vi "main_SMU.vi"() -> ()   [LabVIEW 2018]
uses:
  <instrlib>/Keithley 622x LV 2009/Configure/Source/Typedefs/KE622x -- Voltage Limit.ctl
  <instrlib>/Keithley 622x LV 2009/Configure/Output/Typedefs/KE6221 -- Output Response.ctl
  <instrlib>/Keithley 622x LV 2009/Utility/Typedefs/KE622x -- Instrument Type.ctl
  <instrlib>/Keithley 622x LV 2009/Typedefs/KE622x -- On Off Control.ctl
  <instrlib>/Keithley 622x LV 2009/Configure/Source/Typedefs/KE622x -- Current Range.ctl
  <instrlib>/Keithley 622x LV 2009/Configure/Source/Typedefs/KE622x -- Current Ranges.ctl
  <instrlib>/Keithley 622x LV 2009/Configure/Source/Typedefs/KE622x -- Current Level.ctl
  <vilib>/Utility/file.llb/Write Delimited Spreadsheet (string).vi
  <instrlib>/Keithley 622x LV 2009/Keithley 622x.lvlib
  <instrlib>/Keithley 2450/Keithley 2450.lvlib
panel:
  in  "Compliance Level (0.1)":dbl=0.1
  in  "Output Level (0)":dbl
  out "Voltage":sgl[](array[numeric])
  in  "VISA resource name":refnum<visa-resource-name>
  in  "VISA Switch":refnum<visa-resource-name>="GPIB::6"
  out "Close Channel List":string
  in  "Configurations":enum32{"Radio Selection 1", "Radio Selection 2"}(radio)
  out "Iteration number":i32
  out "Current  (A)":dbl
  out "Mean Voltage  (V1-V8)":dbl
  in  "Step Size":T1=0.001 min=-0.105 max=0.105 format="%.4p"
  in  "End":T1=0.001 min=-0.105 max=0.105 format="%.4p"
  in  "Start":T1=0.001 min=-0.105 max=0.105 format="%.4p"
  in  "Turn Off Output If Voltage Limit?":bool=TRUE
  out "Interlock Tripped?":bool
  out "Voltage Limit?":bool
  in  "Check For SCPI Errors? (T)":bool=TRUE
  in  "Current Range In":T2={"Auto Range?"=TRUE, "Man / Selected\nRange"=enum."2nA"}
  in  "Analog Filter State":T4
  in  "Output Response":T5=enum."Slow"
  in  "Voltage Limit (V)":T6=10.0 min=0.1 max=105.0 step=0.01 format="%.2p"
  out "error at Current off":errorcluster
  out "error at current On":errorcluster
  in  "VISA resource dc ac current source (16)":refnum<visa-resource-name>
  out "Configuration Error":errorcluster
  in  "array":dbl[](array[numeric])
  out "output array":dbl[](array[numeric])
  in  "Instrument Type 2":T7=enum."KE6221"
  # "( select : GPIB0::16::INSTR )"
  # "( select : USB0::0x05E6::0x2450::04345639::INSTR )"
  # "( select : USB0::0x05E6::0x3706::04368238::INSTR )"
types:
  T1 = typedef "Keithley 622x.lvlib/KE622x -- Current Level.ctl" = dbl
  T2 = typedef "Keithley 622x.lvlib/KE622x -- Current Range.ctl" = cluster{"Auto Range?":bool, "Man / Selected\nRange":T3}
  T3 = typedef "Keithley 622x.lvlib/KE622x -- Current Ranges.ctl" = enum16{"2nA", "20nA", "200nA", "2uA", "20uA", "200uA", "2mA", "20mA", "100mA"}
  T4 = typedef "Keithley 622x.lvlib/KE622x -- On Off Control.ctl" = enum16{"Off", "On"}
  T5 = typedef "Keithley 622x.lvlib/KE6221 -- Output Response.ctl" = enum16{"Fast", "Slow"}
  T6 = typedef "Keithley 622x.lvlib/KE622x -- Voltage Limit.ctl" = dbl
  T7 = typedef "Keithley 622x.lvlib/KE622x -- Instrument Type.ctl" = enum16{"KE6220", "KE6221"}
  T8 = enum16{"Close", "Close Exclusive", "Close Slot Exclusive", "Open", "Open All"}
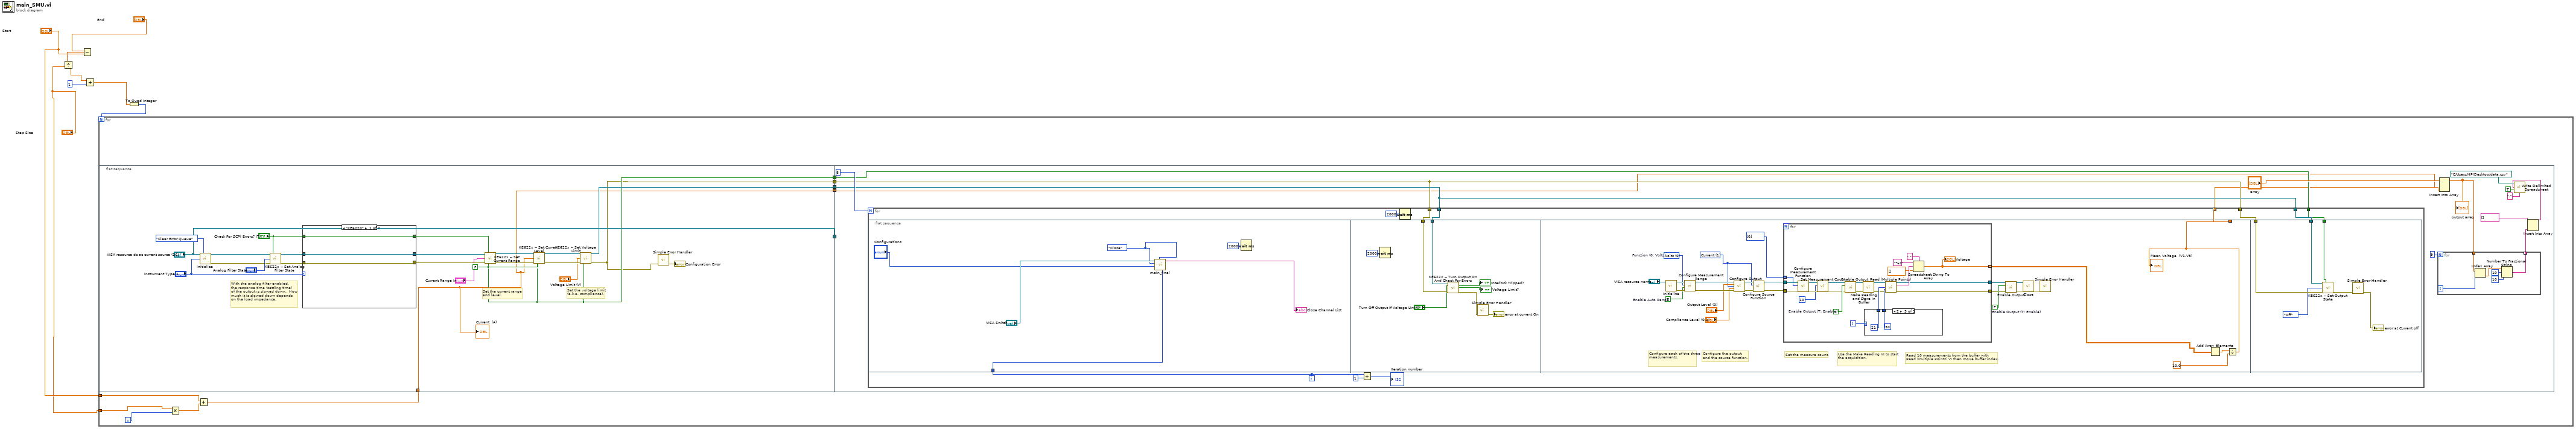
[diagram p0: block diagram]
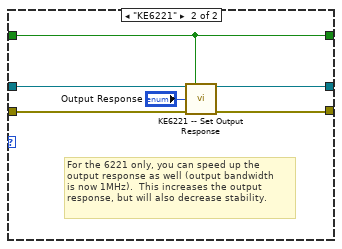
[diagram p2: hidden frame]
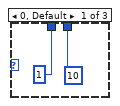
[diagram p3: hidden frame]
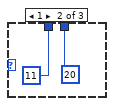
[diagram p4: hidden frame]
diagram:
  n1 = Subtract(x="End", y="Start") -> (x-y=w8:T1)
  n2 = Divide(x=w8, y="Step Size") -> (x/y=w4:T1)
  n3 = Add(x=w4, y=1) -> (x+y=w2:T1)
  n4 = To Quad Integer(1:w2) -> (0:w1:i64)
  n5 = for {
    N: w1 -> [_]
    tunnel: "Step Size" -> [w13]
    tunnel: "Start" -> [w12]
    i -> [w9]
    n6 = flat-sequence {
      tunnel: ["VISA resource dc ac current source (16)"] -> w18
      tunnel: [w22] -> w17
      tunnel: [w20] -> w16
      tunnel: [w21] -> w15
      tunnel: [w19] -> w14
      tunnel: w11 -> [w19]
      tunnel: w18 -> [_]
      tunnel: w17 -> [w63]
      tunnel: w16 -> [w62]
      tunnel: w15 -> [w61]
      tunnel: w14 -> [w51]
      frame #0 {
        w29 = FALSE ("Read Back Set Values? (T)")
        # "Set the voltage limit\n(a.k.a. compliance)."
        # "Set the current range\nand level."
        # "With the analog filter enabled,\nthe response time (settling time)\nof the output is slowed down.  How\nmuch it is slowed down depends\non the load impedance."
        n7 = call <instrlib>:"Initialize.vi"("VISA resource name"="VISA resource dc ac current source (16)", "Error Queue Option"=enum16{"Clear Error Queue", "Error Query"}."Clear Error Queue", "Instrument Type"="Instrument Type 2") -> ("VISA resource name out"=w39:refnum<visa-resource-name>, "error out"=w38:errorcluster)  [unwired: 11 in]
        n8 = call <instrlib>:"KE622x -- Set Analog Filter State.vi"("Resource In"=w39, "Check For SCPI Errors? (T)"="Check For SCPI Errors? (T)", "Analog Filter State"="Analog Filter State", "error in (no error)"=w38) -> ("Resource Out (dupl)"=w37:refnum<visa-resource-name>, "error out"=w35:errorcluster)  [unwired: 10 in]
        n9 = case shown="\"KE6220\"" "Instrument Type 2" {
          tunnel: w37 -> [w43 w50]
          tunnel: w35 -> [w42 w48]
          tunnel: [w43 w47] -> w32
          tunnel: "Check For SCPI Errors? (T)" -> [w44 w46]
          tunnel: [w44 w46] -> w21
          tunnel: [w42 w45] -> w33
          frame "KE6220" {
          }
          frame "KE6221" {
            # "For the 6221 only, you can speed up the\noutput response as well (output bandwidth\nis now 1MHz).  This increases the output\nresponse, but will also decrease stability."
            n10 = call <instrlib>:"KE6221 -- Set Output Response.vi"("Resource In"=w50, "Check For SCPI Errors? (T)"=w46, "KE6221 Output Response"="Output Response", "error in (no error)"=w48) -> ("Resource Out (dupl)"=w47:refnum<visa-resource-name>, "error out"=w45:errorcluster)  [unwired: 10 in]
          }
        }
        n11 = call <instrlib>:"KE622x -- Set Current Range.vi"("Resource In"=w32, "Check For SCPI Errors? (T)"=w21, "Current Range In"="Current Range In", "error in (no error)"=w33, "Read Back Set Values? (T)"=w29) -> ("Resource Out (dupl)"=w31:refnum<visa-resource-name>, "error out"=w30:errorcluster)  [unwired: 8 in, 1 out]
        n12 = call <instrlib>:"KE622x -- Set Current Level.vi"("Resource In"=w31, "Check For SCPI Errors? (T)"=w21, "Current Level (A) In"=w19, "error in (no error)"=w30, "Read Back Set Value? (T)"=w29) -> ("Resource Out (dupl)"=w28:refnum<visa-resource-name>, "error out"=w27:errorcluster)  [unwired: 8 in, 1 out]
        n13 = call <instrlib>:"KE622x -- Set Voltage Limit.vi"("Resource In"=w28, "Check For SCPI Errors? (T)"=w21, "Voltage Limit (V)"="Voltage Limit (V)", "error in (no error)"=w27) -> ("Resource Out (dupl)"=w22:refnum<visa-resource-name>, "error out"=w20:errorcluster)  [unwired: 10 in]
        n14 = call <vilib>:"Simple Error Handler.vi"("error in (no error)"=w20) -> ("error out"=→"Configuration Error":errorcluster)  [unwired: 4 in, 4 out]
        "Current  (A)" <- w19
      }
      frame #1 {
        n15 = for {
          N: 8 -> [_]
          tunnel: [w80] -> w52 mode=indexing
          tunnel: w63 -> [w79]
          tunnel: w62 -> [w78]
          tunnel: w63 -> [w77]
          tunnel: w62 -> [w76]
          tunnel: w61 -> [w75]
          i -> [w73]
          n16 = flat-sequence {
            tunnel: w73 -> [w86]
            tunnel: w79 -> [w95]
            tunnel: w78 -> [w94]
            tunnel: [w119] -> w80
            tunnel: w77 -> [w155]
            tunnel: w76 -> [w154]
            tunnel: w75 -> [w150]
            frame #0 {
              w82 = T8."Close" ("Operation 3")
              n17 = call "main_final.vi"("Numeric"=w86, "Operation 2"=w82, "Radio Buttons"="Configurations", "Operation 3"=w82, "VISA Refnum in"="VISA Switch") -> ("Close Channel List 2"=→"Close Channel List":string)  [unwired: 6 in]
              n18 = Wait (ms)(milliseconds to wait=u32 2000) -> ()  [unwired: 1 out]
            }
            frame #1 {
              n19 = Wait (ms)(milliseconds to wait=u32 2000) -> ()  [unwired: 1 out]
              n20 = call <instrlib>:"KE622x -- Turn Output On And Check For Errors.vi"("Resource In"=w95, "Turn Off Output If Compliance?"="Turn Off Output If Voltage Limit?", "error in (no error)"=w94) -> ("Interlock Tripped?"=→"Interlock Tripped?":bool, "Compliance?"=→"Voltage Limit?":bool, "error out"=w89:errorcluster)  [unwired: 9 in, 1 out]
              n21 = call <vilib>:"Simple Error Handler.vi"("error in (no error)"=w89) -> ("error out"=→"error at current On":errorcluster)  [unwired: 4 in, 4 out]
            }
            frame #2 {
              w98 = u16 1 items=["Voltage", "Current"] ("Source Mode  (0: Voltage)")
              w110 = FALSE  # Enable Output (T: Enable)
              w113 = u16 0 items=["Volts", "Current", "Resistance"]  # Function (0: Volts)
              w114 = TRUE  # Enable Auto Range
              # "Read 10 measurements from the buffer with \nRead (Multiple Points) VI then move buffer index."
              # "Set the measure count."
              # "Use the Make Reading VI to start the acquisition."
              # "Configure the output \nand the source function."
              # "Configure each of the three measurements."
              n22 = call <instrlib>:"Initialize.vi"("VISA resource name"="VISA resource name") -> ("error out"=w115:errorcluster, "VISA resource name out"=w116:refnum<visa-resource-name>)  [unwired: 9 in]
              n23 = call <instrlib>:"Configure Measurement Range.vi"("error in (no error)"=w115, "Enable Auto Range (T:Enable)"=w114, "Function (0: Volts)"=w113, "VISA resource name"=w116) -> ("error out"=w108:errorcluster, "VISA resource name out"=w109:refnum<visa-resource-name>)  [unwired: 6 in]
              n24 = call <instrlib>:"Configure Output.vi"("VISA resource name"=w109, "Source Level (0)"="Output Level (0)", "Source Mode  (0: Voltage)"=w98, "Source Limit Level (0.1)"="Compliance Level (0.1)", "error in (no error)"=w108) -> ("VISA resource name out"=w104:refnum<visa-resource-name>, "error out"=w105:errorcluster)  [unwired: 9 in]
              n25 = call <instrlib>:"Configure Source Function.vi"("error in (no error)"=w105, "Function (0: Volts)"=w98, "VISA resource name"=w104) -> ("error out"=w102:errorcluster, "VISA resource name out"=w103:refnum<visa-resource-name>)  [unwired: 7 in]
              n26 = for {
                tunnel: [w133] -> w107
                tunnel: [w132] -> w106
                tunnel: w102 -> [w143]
                tunnel: w103 -> [w142]
                tunnel: u16[] [0] -> [w141] mode=indexing
                tunnel: [w121] -> w97 mode=indexing
                i -> [w129]
                w126 = TRUE  # Enable Output (T: Enable)
                n27 = call <instrlib>:"Configure Measurement Function.vi"("error in (no error)"=w143, "Function (0: Volts)"=w141, "VISA resource name"=w142) -> ("error out"=w140:errorcluster, "VISA resource name out"=w139:refnum<visa-resource-name>)  [unwired: 7 in]
                n28 = call <instrlib>:"Set Measurement Count.vi"("error in (no error)"=w140, "Measurement Count (1)"=u32 10 ("millisecond multiple"), "VISA resource name"=w139) -> ("error out"=w124:errorcluster, "VISA resource name out"=w125:refnum<visa-resource-name>)  [unwired: 7 in]
                n29 = call <instrlib>:"Enable Output.vi"("error in (no error)"=w124, "Enable Output (T: Enable)"=w126, "VISA resource name"=w125) -> ("error out"=w122:errorcluster, "VISA resource name out"=w123:refnum<visa-resource-name>)  [unwired: 7 in]
                n30 = call <instrlib>:"Make Reading and Store in Buffer.vi"("VISA resource name"=w123, "error in (no error)"=w122) -> ("VISA resource name out"=w128:refnum<visa-resource-name>, "error out"=w127:errorcluster)  [unwired: 12 in]
                n31 = case shown="2" w129 {
                  tunnel: [u32 1 ("millisecond multiple") u32 11 ("millisecond multiple") u32 21 ("millisecond multiple")] -> w131
                  tunnel: [u32 10 ("millisecond multiple") u32 20 ("millisecond multiple") u32 30 ("millisecond multiple")] -> w130
                  frame 0, Default {
                  }
                  frame 1 {
                  }
                  frame 2 {
                  }
                }
                n32 = call <instrlib>:"Read (Multiple Points).vi"("VISA resource name"=w128, "Start Index (1)"=w131, "End Index (1)"=w130, "error in (no error)"=w127) -> ("VISA resource name out"=w133:refnum<visa-resource-name>, "Data out"=w137:string, "error out"=w132:errorcluster)  [unwired: 9 in]
                n33 = Spreadsheet String To Array(delimiter (Tab)=",", format string="%s", spreadsheet string=w137, array type (2D Dbl)=dbl[] []) -> (array=w121:dbl[])
                "Voltage" <- w121
              }
              n34 = call <instrlib>:"Enable Output.vi"("error in (no error)"=w106, "Enable Output (T: Enable)"=w110, "VISA resource name"=w107) -> ("error out"=w111:errorcluster, "VISA resource name out"=w112:refnum<visa-resource-name>)  [unwired: 7 in]
              n35 = call <instrlib>:"Close.vi"("error in (no error)"=w111, "VISA resource name"=w112) -> ("error out"=w118:errorcluster)  [unwired: 9 in]
              n36 = call <vilib>:"Simple Error Handler.vi"("error in (no error)"=w118) -> ()  [unwired: 4 in, 5 out]
              n37 = Add Array Elements(numeric array=w97) -> (sum=w120:dbl)
              n38 = Divide(x=w120, y=10.0) -> (x/y=w119:dbl)
              "Mean Voltage  (V1-V8)" <- w119
            }
            frame #3 {
              n39 = call <instrlib>:"KE622x -- Set Output State.vi"("Resource In"=w155, "Check For SCPI Errors? (T)"=w150, "Output State"=KE622x_--_On_Off_Control."Off", "error in (no error)"=w154) -> ("error out"=w151:errorcluster)  [unwired: 10 in, 1 out]
              n40 = call <vilib>:"Simple Error Handler.vi"("error in (no error)"=w151) -> ("error out"=→"error at Current off":errorcluster)  [unwired: 4 in, 4 out]
            }
          }
          n41 = Add(x=w73, y=1) -> (x+y=→"Iteration number":i32)
          n42 = Wait (ms)(milliseconds to wait=u32 2000) -> ()  [unwired: 1 out]
        }
        n43 = Insert Into Array(array="array", new element #1=w51, new element #2=w52) -> (w57:dbl[])  [unwired: 1 in]
        "output array" <- w57
        n44 = for {
          N: 9 -> [_]
          tunnel: w57 -> [w71]
          tunnel: [w68] -> w56 mode=indexing
          i -> [w70]
          n45 = Index Array(array=w71, index=w70) -> (element=w69:dbl)
          n46 = Number To Fractional String(number=w69, width (-)=i16 10, precision (6)=i16 10) -> (F-format string=w68:string)  [unwired: 1 in]
        }
        n47 = Insert Into Array(array=string[] [], new element=w56) -> (w54:string[])  [unwired: 1 in]
        n48 = call-poly <vilib>:"Write Delimited Spreadsheet.vi"("file path (dialog if empty)"=path "C:/Users/HP/Desktop/data.csv", "1D data"=w54, "append to file? (new file:F)"=TRUE, "delimiter (\\t)"="," ("delimiter (\\t)")) -> ()  [unwired: 10 in, 2 out]
      }
    }
    n49 = Multiply(x=w13, y=w9) -> (x*y=w10:T1)
    n50 = Add(x=w12, y=w10) -> (x+y=w11:T1)
  }
